vi "_mzData Spectrum.vi"(5 "Spectrum":i32[](array[numeric]), 6 "FixedMass (amu)":dbl, 7 "id":i32=1) -> (3 "Output XML":string)   [LabVIEW 2012]
uses:
  Configuration/_Global Configuration.vi
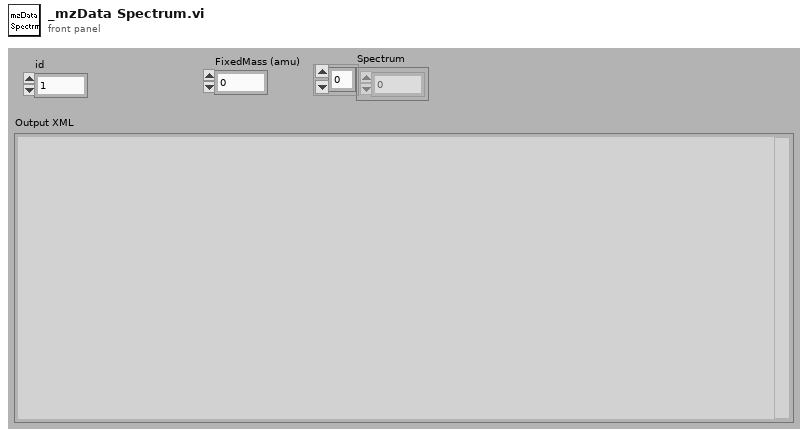
[diagram p1: front panel]
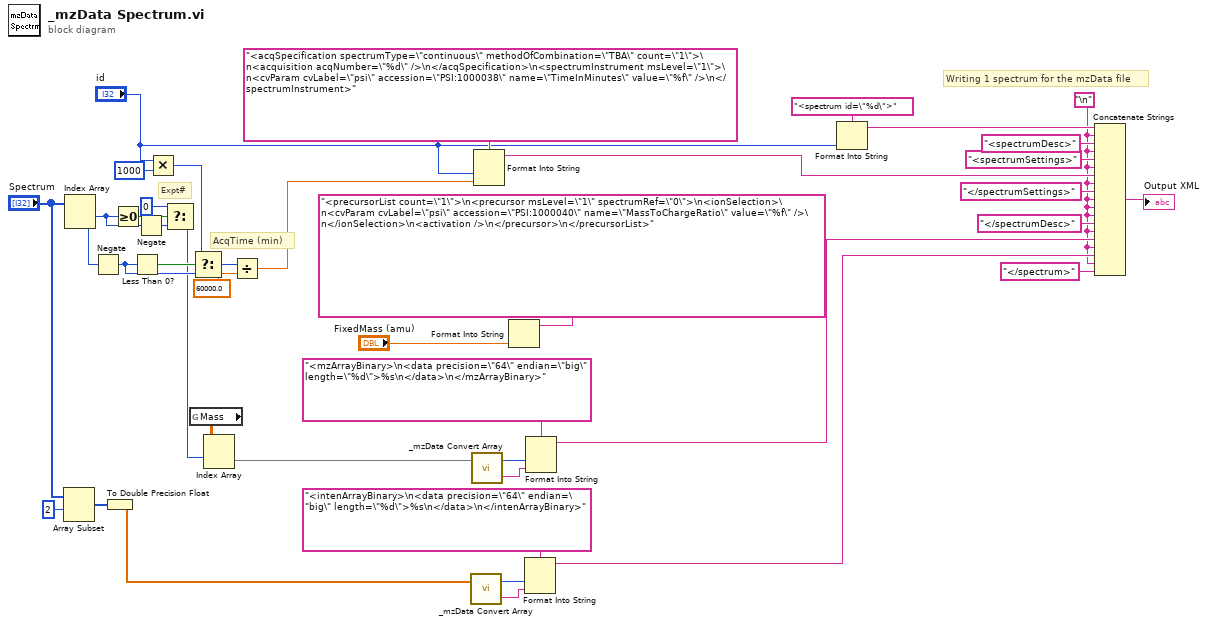
[diagram p0: block diagram]
diagram:
  w4 = "\n"
  # "AcqTime (min)"
  # "Expt#"
  # "Writing 1 spectrum for the mzData file"
  n1 = Array Subset(array="Spectrum", index=2) -> (w14:i32[])  [unwired: 1 in]
  n2 = Index Array(array="Spectrum") -> (element #1=w28:i32, element #2=w25:i32)  [unwired: 2 in]
  n3 = Negate(x=w25) -> (-x=w23:i32)
  n4 = To Double Precision Float(number=w14) -> (double precision float=w6:dbl[])
  n5 = Greater Or Equal To 0?(x=w28) -> (x >= 0?=w29:bool)
  n6 = Less Than 0?(x=w23) -> (x < 0?=w24:bool)
  n7 = Negate(x=w28) -> (-x=w27:i32)
  n8 = Multiply(x="id", y=1000) -> (x*y=w21:i32)
  n9 = Select(t=0, s=w29, f=w27) -> (s? t:f=w15:i32)
  n10 = global read "_Global Configuration.vi" "Mass"() -> (w16:dbl[][])
  n11 = Select(t=w21, s=w24, f=w23) -> (s? t:f=w20:i32)
  n12 = Index Array(array=w16, index (row)=w15) -> (element=w1:dbl[])  [unwired: 1 in]
  n13 = Divide(x=w20, y=60000.0) -> (x/y=w3:dbl)
  n14 = call "_mzData Convert Array.vi"("Array"=w6) -> ("String"=w9:string, "Length"=w8:i32)  [unwired: 1 out]
  n15 = call "_mzData Convert Array.vi"("Array"=w1) -> ("String"=w11:string, "Length"=w12:i32)  [unwired: 1 out]
  n16 = Format Into String(format string="<acqSpecification spectrumType=\"continuous\" methodOfCombination=\"TBA\" count=\"1\">\n<acquisition acqNumber=\"%d\" />\n</acqSpecification>\n<spectrumInstrument msLevel=\"1\">\n<cvParam cvLabel=\"psi\" accession=\"PSI:1000038\" name=\"TimeInMinutes\" value=\"%f\" />\n</spectrumInstrument>", "id", w3) -> (resulting string=w34:string)  [unwired: 2 in, 1 out]
  n17 = Format Into String(format string="<precursorList count=\"1\">\n<precursor msLevel=\"1\" spectrumRef=\"0\">\n<ionSelection>\n<cvParam cvLabel=\"psi\" accession=\"PSI:1000040\" name=\"MassToChargeRatio\" value=\"%f\" />\n</ionSelection>\n<activation />\n</precursor>\n</precursorList>", "FixedMass (amu)") -> ()  [unwired: 2 in, 2 out]
  n18 = Format Into String(format string="<intenArrayBinary>\n<data precision=\"64\" endian=\"big\" length=\"%d\">%s\n</data>\n</intenArrayBinary>", w8, w9) -> (resulting string=w5:string)  [unwired: 2 in, 1 out]
  n19 = Format Into String(format string="<mzArrayBinary>\n<data precision=\"64\" endian=\"big\" length=\"%d\">%s\n</data>\n</mzArrayBinary>", w12, w11) -> (resulting string=w10:string)  [unwired: 2 in, 1 out]
  n20 = Format Into String(format string="<spectrum id=\"%d\">", "id") -> (resulting string=w36:string)  [unwired: 2 in, 1 out]
  n21 = Concatenate Strings(w36, w4, "<spectrumDesc>", w4, "<spectrumSettings>", w4, w34, w4, "</spectrumSettings>", w4, w4, w4, "</spectrumDesc>", w4, w10, w4, w5, w4, "</spectrum>") -> (→"Output XML":string)
